vi "Processing Reference (FPGA).vi"() -> ()   [LabVIEW 2019]
uses:
  <vilib>/Platform/TimedLoop/XDataNode/wakeup.ctl
  <vilib>/Platform/TimedLoop/XDataNode/XDNodeRunTimeDep.lvlib
  <vilib>/Platform/TimedLoop/XDataNode/nitl_modes.ctl
  <vilib>/Platform/TimedLoop/XDataNode/timing_clust.ctl
  <vilib>/Platform/TimedLoop/XDataNode/XDataNode.xnode
  <vilib>/eio/EIONode/EIONode.xnode
  <instrlib>/_niInstr/Basic Elements/v1/FPGA/niInstr Basic Elements v1 FPGA.lvlib
  <instrlib>/_niInstr/Data Formatting/v1/FPGA/niInstr Data Formatting v1 FPGA.lvlib
  <vilib>/rvi/DataTransferAndStorage/Container/XNode/niFpgaContainer.xnode
  <vilib>/rvi/FIFO/Fifo_Resource/nirvififoEmulationWrite.vi
  <vilib>/rvi/FIFO/Fifo_Resource/nirvififoEmulationRead.vi
  <vilib>/rvi/LocalResourceManager/LocalResourceManager.xnode
  <vilib>/rvi/FIFO/Fifo_Resource/nirvififoEmulationGetNumberOfElementsToRead.vi
  <vilib>/rvi/interface/RandomDataEmulation/nirviRandomDataFpgaMultiElementTemplate.vi
  <instrlib>/_niInstr/Data Formatting/v1/FPGA/Private/Convert/U8 array to Boolean Array.vi
  <instrlib>/_niInstr/Data Formatting/v1/FPGA/Private/Convert/Boolean Array to U8 Array.vi
  <vilib>/rvi/eio/common/nirviEmuTemplateMethod_errors.vi
  <instrlib>/_niInstr/Basic Elements/v1/FPGA/Private/Count Up U32.vi
  <instrlib>/_niInstr/Basic Elements/v1/FPGA/Private/Count Down U16.vi
  <instrlib>/_niInstr/Basic Elements/v1/FPGA/Private/Count Up U8.vi
  <vilib>/rvi/DataTransferAndStorage/Container/Common/niFpgaContainerGetUniqueNameForEmu.vi
  <vilib>/rvi/DataTransferAndStorage/Container/Common/niFpgaContainerSetEmuInfo.vi
  <vilib>/rvi/eio/common/nirviEmuReportErrorAndStop.vi
  <instrlib>/_niInstr/Instruction Framework/v1/FPGA/Interfaces/Address Space/Address Space Instruction.ctl
  <instrlib>/_niInstr/Instruction Framework/v1/FPGA/Interfaces/Address Space/Address Space.lvclass
  <instrlib>/_niInstr/Instruction Framework/v1/FPGA/Typedefs/Response.ctl
  <instrlib>/_niInstr/Instruction Framework/v1/FPGA/Typedefs/niInstr Instruction Framework v1 FPGA.lvlib
panel:
  out "AXI response out":T1
  out "ready for input":bool
  out "done":bool
  in  "AXI instruction in":T2
  out "channel status":T3(array[cluster])
  out "rx fifo overflow":bool[](array[boolean])
  out "data out port 4":u8[](array[numeric])
  out "data out port 5":u8[](array[numeric])
  in  "data in port 4":u8[](array[numeric])=[0, 0, 0, 0, 0, 0, 0, 0, 0, 0, 0, 0, 0, 0, 0, 0, 0, 0, 0, 0, 0, 0, 0, 0, 0, 0, 0, 0, 0, 0, 0, 0]
  in  "data in port 5":u8[](array[numeric])=[0, 0, 0, 0, 0, 0, 0, 0, 0, 0, 0, 0, 0, 0, 0, 0, 0, 0, 0, 0, 0, 0, 0, 0, 0, 0, 0, 0, 0, 0, 0, 0]
  in  "rx fifo overflow clear":bool
  in  "reset falling edge detect":bool
  out "falling edge detected":bool
  in  "ignore rx fifo prime depth":bool[](array[boolean])=[TRUE, TRUE, TRUE, TRUE, TRUE, TRUE]
  in  "acq length":u16
  in  "software trigger":bool
  in  "data in port 3":u8[](array[numeric])=[0, 0, 0, 0, 0, 0, 0, 0, 0, 0, 0, 0, 0, 0, 0, 0, 0, 0, 0, 0, 0, 0, 0, 0, 0, 0, 0, 0, 0, 0, 0, 0]
  in  "data in port 2":u8[](array[numeric])=[0, 0, 0, 0, 0, 0, 0, 0, 0, 0, 0, 0, 0, 0, 0, 0, 0, 0, 0, 0, 0, 0, 0, 0, 0, 0, 0, 0, 0, 0, 0, 0]
  out "data out port 2":u8[](array[numeric])
  out "data out port 3":u8[](array[numeric])
  in  "tx fifo overflow clear":bool
  out "rx fifo fullness":u32[](array[numeric])
  out "tx fifo overflow":bool[](array[boolean])
  in  "write data":bool
  out "read fifos":bool
  in  "reset read fifo":bool
  in  "rx fifo prime depth":u32=10
  in  "use counter":bool
  in  "data in port 1":u8[](array[numeric])=[0, 0, 0, 0, 0, 0, 0, 0, 0, 0, 0, 0, 0, 0, 0, 0, 0, 0, 0, 0, 0, 0, 0, 0, 0, 0, 0, 0, 0, 0, 0, 0]
  in  "data in port 0":u8[](array[numeric])=[0, 0, 0, 0, 0, 0, 0, 0, 0, 0, 0, 0, 0, 0, 0, 0, 0, 0, 0, 0, 0, 0, 0, 0, 0, 0, 0, 0, 0, 0, 0, 0]
  out "data out port 1":u8[](array[numeric])
  out "data out port 0":u8[](array[numeric])
  out "clocks valid":bool[](array[boolean])
  out "user clk":u32
  out "status.mgt ref clocks locked":bool
  out "status.mgt ref clock valid":bool
  out "status.config complete":bool
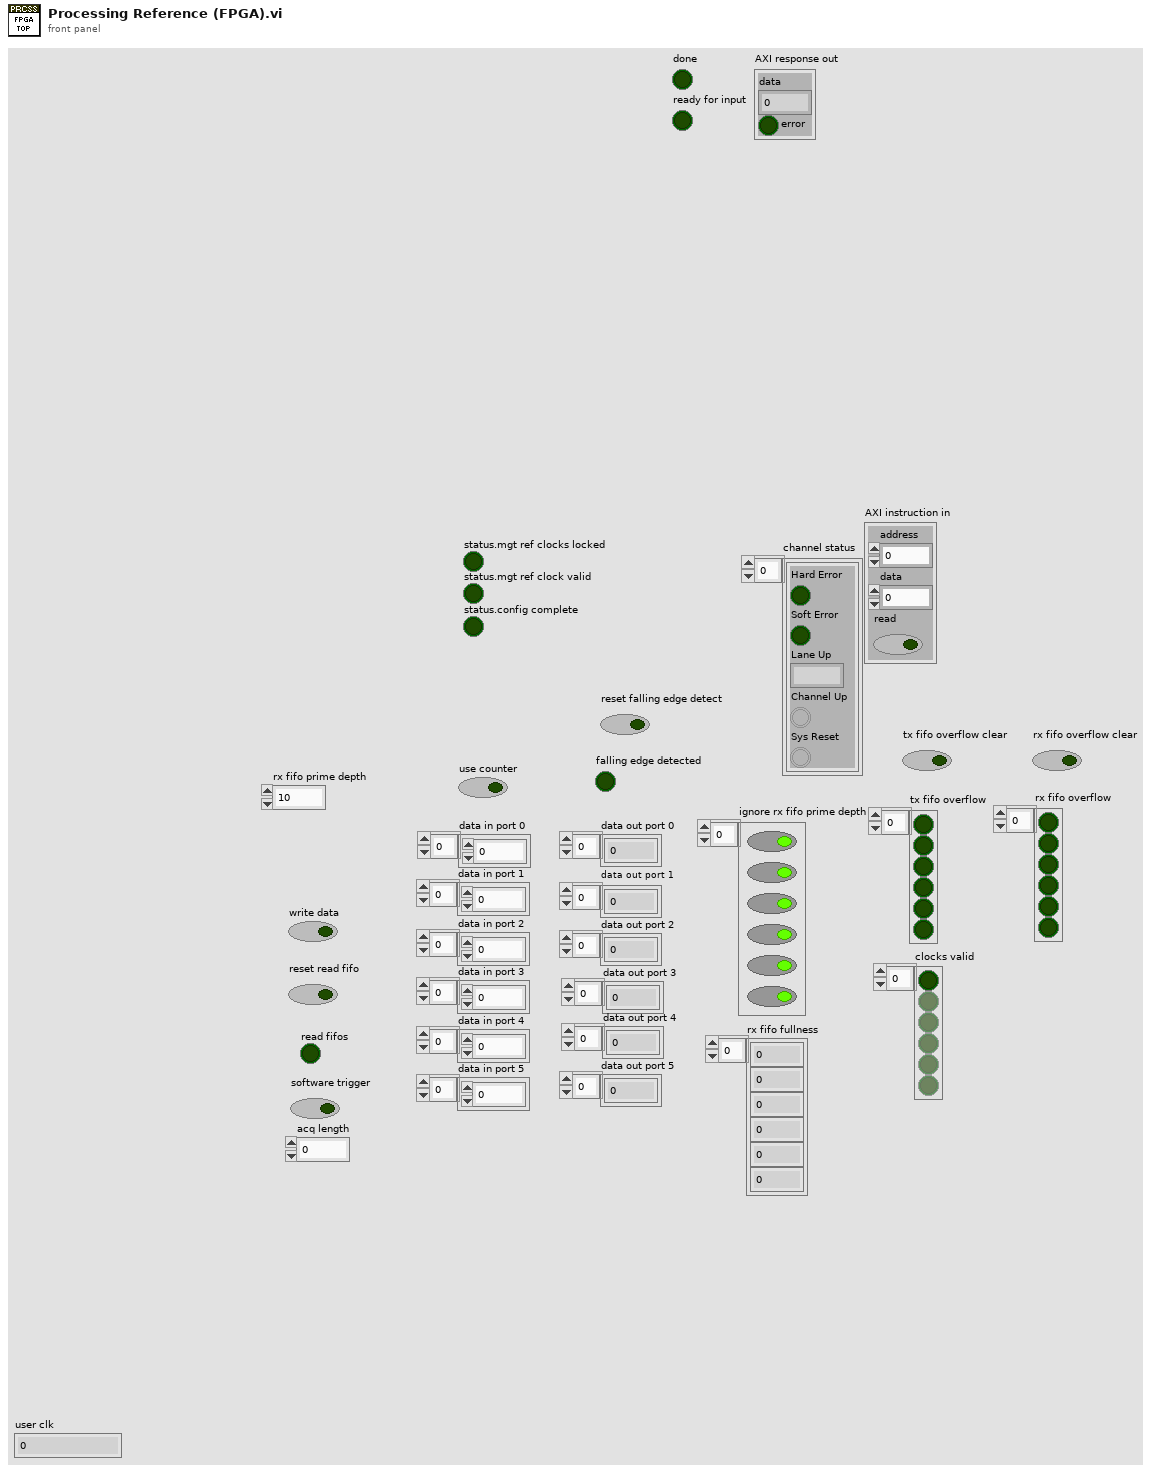
[diagram p1: front panel]
types:
  T1 = typedef "niInstr Instruction Framework v1 FPGA.lvlib/Response.ctl" = cluster{"data":u64, "error":bool}
  T2 = typedef "niInstr Instruction Framework Interfaces v1 FPGA.lvlib/Address Space.lvclass/Address Space Instruction.ctl" = cluster{"address":u32, "data":u64, "read":bool}
  T3 = cluster{"Hard Error":bool, "Soft Error":bool, "Lane Up":fxp<+,4,4>, "Channel Up":bool, "Sys Reset":bool}[]
  T4 = cluster{"m_axis_tvalid":refnum<k21>, "m_axis_tdata_0":refnum<k21>, "m_axis_tdata_1":refnum<k21>, "m_axis_tdata_2":refnum<k21>, "m_axis_tdata_3":refnum<k21>}
  T5 = cluster{"s_axis_tvalid":refnum<k21>, "s_axis_tdata_0":refnum<k21>, "s_axis_tdata_1":refnum<k21>, "s_axis_tdata_2":refnum<k21>, "s_axis_tdata_3":refnum<k21>, "s_axis_tready":refnum<k21>}
  T6 = typedef "XDNodeRunTimeDep.lvlib/timing_clust.ctl" = cluster{"Expected End [f-1]":u64, "Actual End [f-1]":u64, "Finished Late? [f-1]":bool, "Expected End [i-1]":u64, "Actual End [i-1]":u64, "Finished Late? [i-1]":bool, "Expected Start [i]":u64, "Actual Start [i]":u64, "Expected Start [f]":u64, "Actual Start [f]":u64, "Source Name":string, "Structure Name":string, "Period":i64, "Deadline":i64, "Offset":i64, "Start":i64, "Priority":i32, "Timeout":i32, "Mode":T7, "Wakeup Reason":T8, "Error":errorcluster, "Source Type":string, "Secondary Source Type":string, "Global End Time":u64, "Global Start Time":u64, "Frame Duration":u64, "Iteration Duration":u64, "Assigned CPU":i32, "I/O Scan Engine Mode":u32}
  T7 = typedef "XDNodeRunTimeDep.lvlib/nitl_modes.ctl" = enum32{"No Change", "Process missed periods, maintain original phase", "Discard missed periods, maintain original phase", "Process missed periods, ignore original phase", "Discard missed periods, ignore original phase"}
  T8 = typedef "XDNodeRunTimeDep.lvlib/wakeup.ctl" = enum32{"Normal", "Aborted", "Asynchronous wakeup", "Timing source error", "Timed loop error", "Timeout"}
  T9 = typedef "AXI4-Stream Reader FXP64x4 Resources.ctl" = cluster{"AXI4-Stream Reader Resources":cluster{"Use TREADY":bool, "Use TLAST":bool, "TLAST":refnum<k21>, "TREADY":refnum<k21>, "TVALID":refnum<k21>, "Use TKEEP":bool, "Use TSTRB":bool, "Use TUSER":bool}, "TDATA Resources":cluster{"TDATA_0":refnum<k21>, "TDATA_1":refnum<k21>, "TDATA_2":refnum<k21>, "TDATA_3":refnum<k21>}, "TKEEP":refnum<k21>, "TSTRB":refnum<k21>}
  T10 = typedef "AXI4-Stream Writer FXP64x4 Resources.ctl" = cluster{"Writer Resources":cluster{"Use TREADY":bool, "Use TLAST":bool, "TLAST":refnum<k21>, "TREADY":refnum<k21>, "TVALID":refnum<k21>, "Use TSTRB":bool, "Use TKEEP":bool, "Use TUSER":bool}, "TDATA Resources":cluster{"TDATA_0":refnum<k21>, "TDATA_1":refnum<k21>, "TDATA_2":refnum<k21>, "TDATA_3":refnum<k21>}, "TKEEP":refnum<k21>, "TSTRB":refnum<k21>}
  T11 = cluster{"Hard Error":refnum<k21>, "Soft Error":refnum<k21>, "Lane Up":refnum<k21>, "Channel Up":refnum<k21>, "Sys Reset":refnum<k21>}
  T12 = cluster{"Hard Error":bool, "Soft Error":bool, "Lane Up":fxp<+,4,4>, "Channel Up":bool, "Sys Reset":bool}
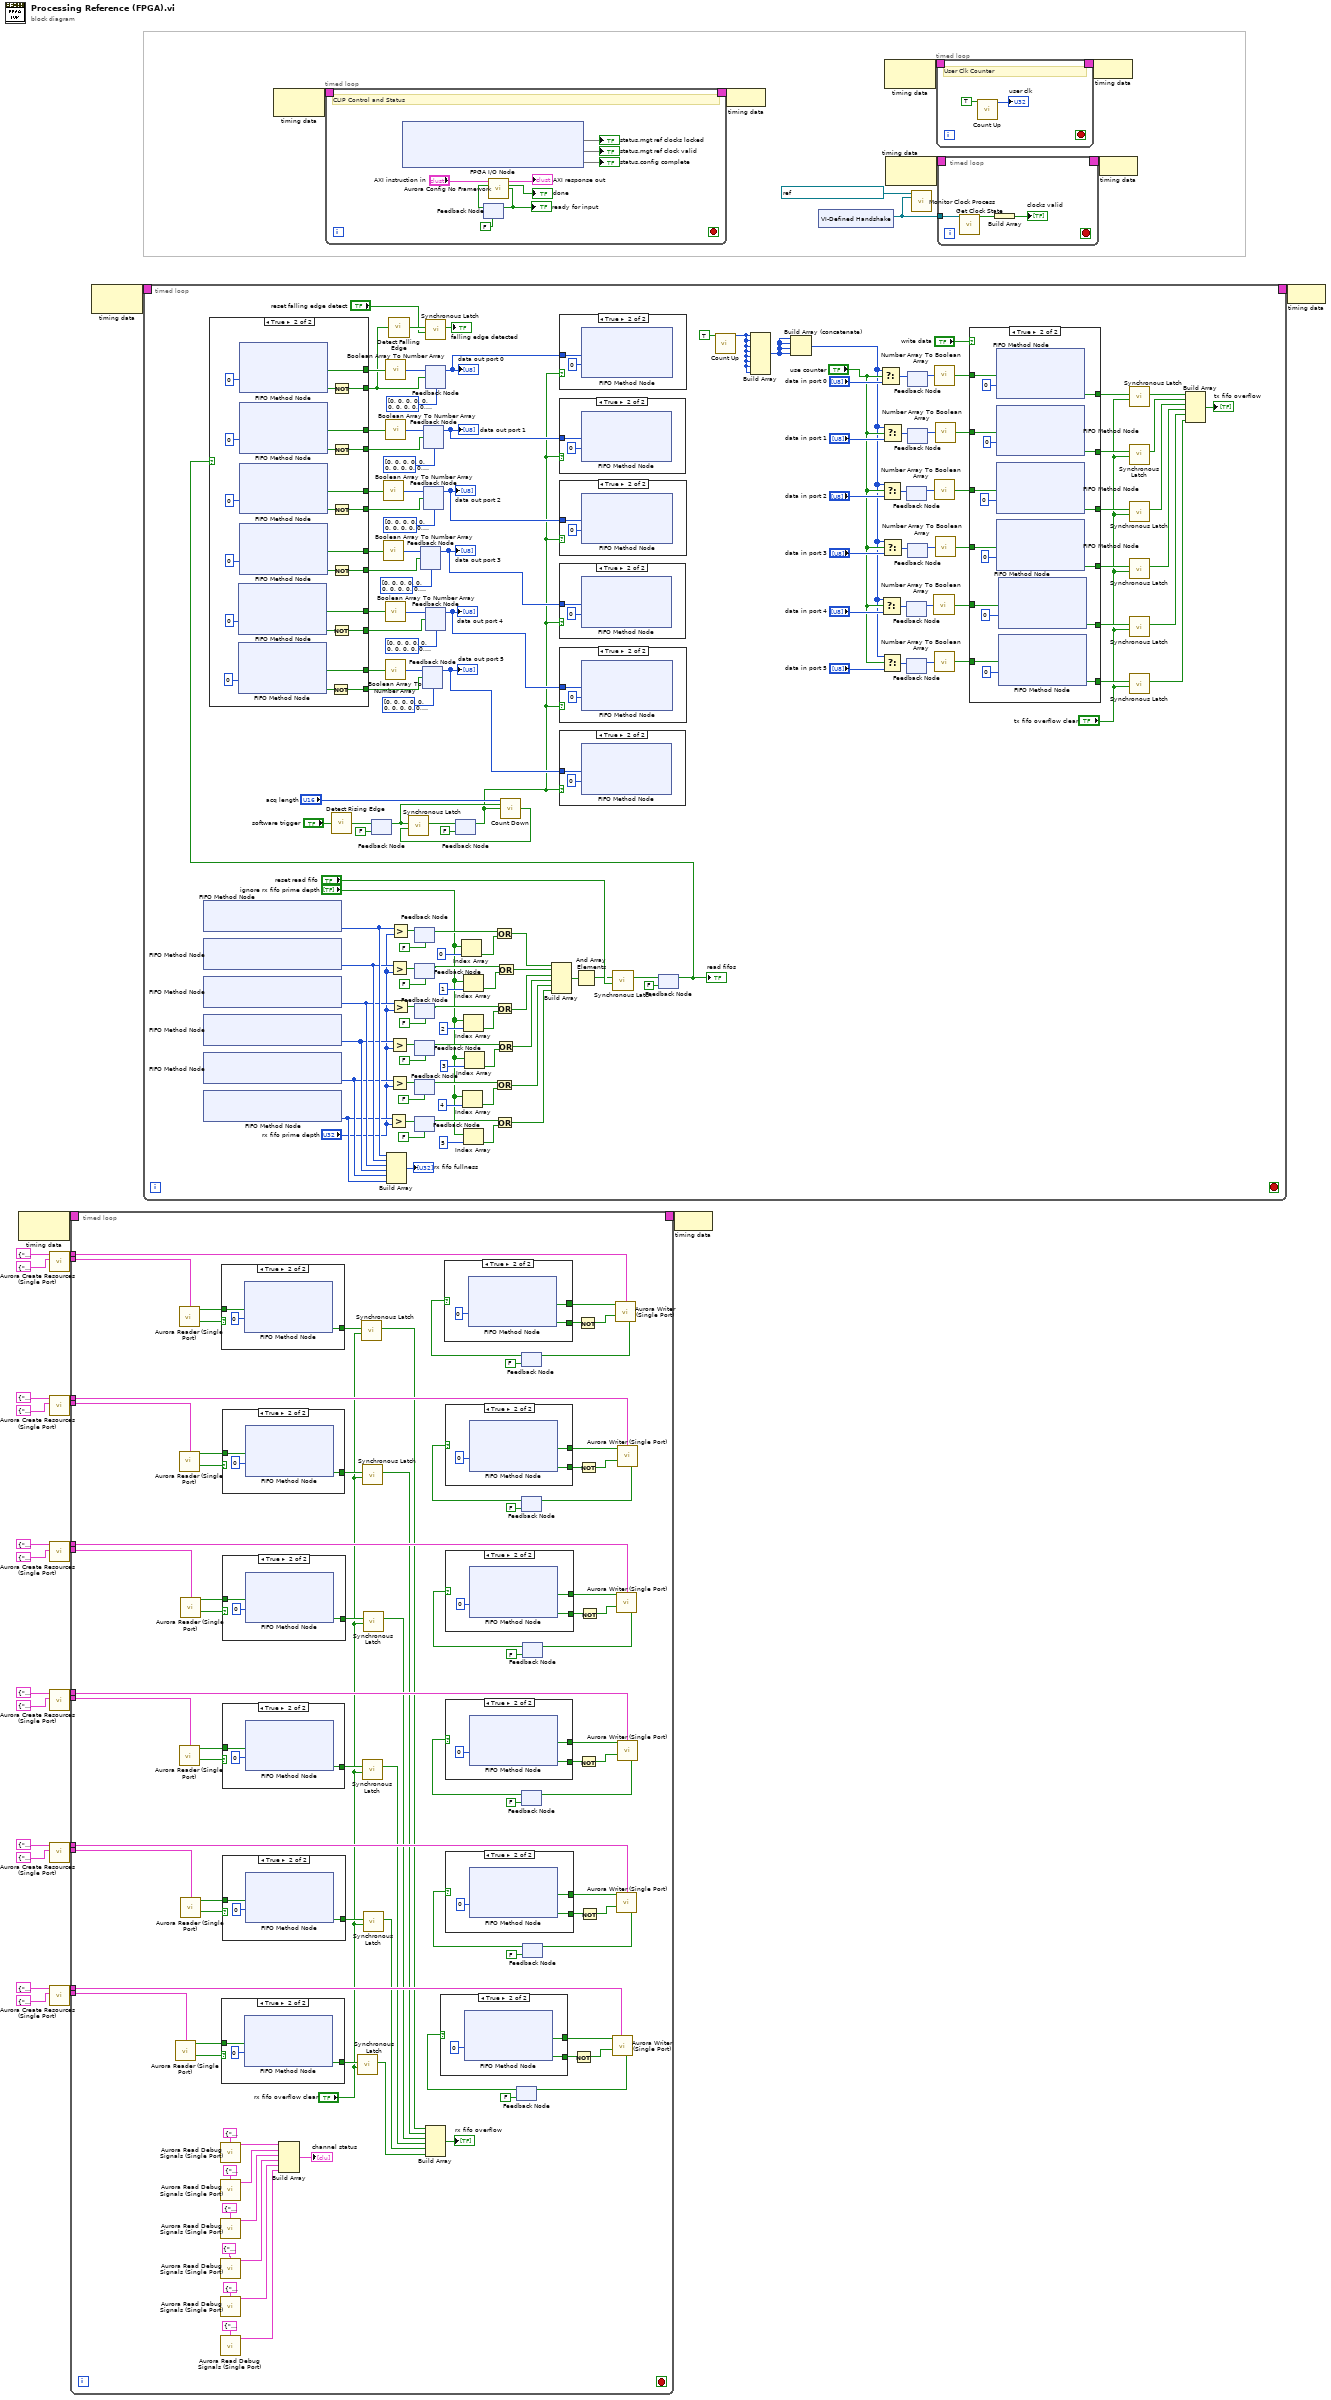
[diagram p0: block diagram]
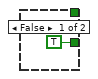
[diagram p2: hidden frame]
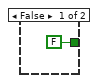
[diagram p3: hidden frame]
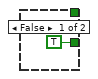
[diagram p4: hidden frame]
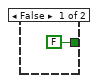
[diagram p5: hidden frame]
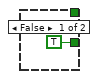
[diagram p6: hidden frame]
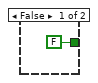
[diagram p7: hidden frame]
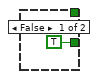
[diagram p8: hidden frame]
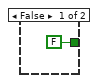
[diagram p9: hidden frame]
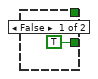
[diagram p10: hidden frame]
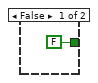
[diagram p11: hidden frame]
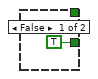
[diagram p12: hidden frame]
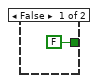
[diagram p13: hidden frame]
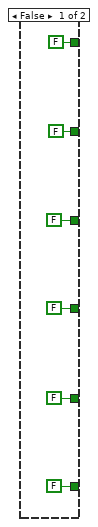
[diagram p20: hidden frame]
diagram:
  n1 = node-c288() -> (w22:T6)  [unwired: 1 in]
  n2 = call "Aurora Create Resources (Single Port).vi"("RX CLIP Resources"=T4 {"m_axis_tvalid"="7902R IO Socket\\uPort0_m_axi_rx_tvalid", "m_axis_tdata_0"="7902R IO Socket\\uPort0_m_axi_rx_tdata_0", "m_axis_tdata_1"="7902R IO Socket\\uPort0_m_axi_rx_tdata_1", "m_axis_tdata_2"="7902R IO Socket\\uPort0_m_axi_rx_tdata_2", "m_axis_tdata_3"="7902R IO Socket\\uPort0_m_axi_rx_tdata_3"}, "TX CLIP Resources"=T5 {"s_axis_tvalid"="7902R IO Socket\\uPort0_s_axi_tx_tvalid", "s_axis_tdata_0"="7902R IO Socket\\uPort0_s_axi_tx_tdata_0", "s_axis_tdata_1"="7902R IO Socket\\uPort0_s_axi_tx_tdata_1", "s_axis_tdata_2"="7902R IO Socket\\uPort0_s_axi_tx_tdata_2", "s_axis_tdata_3"="7902R IO Socket\\uPort0_s_axi_tx_tdata_3", "s_axis_tready"="7902R IO Socket\\uPort0_s_axi_tx_tready"}) -> ("AXI4-Stream Reader FXP64x4"=w20:T9, "AXI4-Stream Writer FXP64x4"=w19:T10)  [unwired: 8 in]
  n3 = call "Aurora Create Resources (Single Port).vi"("RX CLIP Resources"=T4 {"m_axis_tvalid"="7902R IO Socket\\uPort1_m_axi_rx_tvalid", "m_axis_tdata_0"="7902R IO Socket\\uPort1_m_axi_rx_tdata_0", "m_axis_tdata_1"="7902R IO Socket\\uPort1_m_axi_rx_tdata_1", "m_axis_tdata_2"="7902R IO Socket\\uPort1_m_axi_rx_tdata_2", "m_axis_tdata_3"="7902R IO Socket\\uPort1_m_axi_rx_tdata_3"}, "TX CLIP Resources"=T5 {"s_axis_tvalid"="7902R IO Socket\\uPort1_s_axi_tx_tvalid", "s_axis_tdata_0"="7902R IO Socket\\uPort1_s_axi_tx_tdata_0", "s_axis_tdata_1"="7902R IO Socket\\uPort1_s_axi_tx_tdata_1", "s_axis_tdata_2"="7902R IO Socket\\uPort1_s_axi_tx_tdata_2", "s_axis_tdata_3"="7902R IO Socket\\uPort1_s_axi_tx_tdata_3", "s_axis_tready"="7902R IO Socket\\uPort1_s_axi_tx_tready"}) -> ("AXI4-Stream Reader FXP64x4"=w9:T9, "AXI4-Stream Writer FXP64x4"=w10:T10)  [unwired: 8 in]
  n4 = call "Aurora Create Resources (Single Port).vi"("RX CLIP Resources"=T4 {"m_axis_tvalid"="7902R IO Socket\\uPort2_m_axi_rx_tvalid", "m_axis_tdata_0"="7902R IO Socket\\uPort2_m_axi_rx_tdata_0", "m_axis_tdata_1"="7902R IO Socket\\uPort2_m_axi_rx_tdata_1", "m_axis_tdata_2"="7902R IO Socket\\uPort2_m_axi_rx_tdata_2", "m_axis_tdata_3"="7902R IO Socket\\uPort2_m_axi_rx_tdata_3"}, "TX CLIP Resources"=T5 {"s_axis_tvalid"="7902R IO Socket\\uPort2_s_axi_tx_tvalid", "s_axis_tdata_0"="7902R IO Socket\\uPort2_s_axi_tx_tdata_0", "s_axis_tdata_1"="7902R IO Socket\\uPort2_s_axi_tx_tdata_1", "s_axis_tdata_2"="7902R IO Socket\\uPort2_s_axi_tx_tdata_2", "s_axis_tdata_3"="7902R IO Socket\\uPort2_s_axi_tx_tdata_3", "s_axis_tready"="7902R IO Socket\\uPort2_s_axi_tx_tready"}) -> ("AXI4-Stream Reader FXP64x4"=w7:T9, "AXI4-Stream Writer FXP64x4"=w8:T10)  [unwired: 8 in]
  n5 = call "Aurora Create Resources (Single Port).vi"("RX CLIP Resources"=T4 {"m_axis_tvalid"="7902R IO Socket\\uPort3_m_axi_rx_tvalid", "m_axis_tdata_0"="7902R IO Socket\\uPort3_m_axi_rx_tdata_0", "m_axis_tdata_1"="7902R IO Socket\\uPort3_m_axi_rx_tdata_1", "m_axis_tdata_2"="7902R IO Socket\\uPort3_m_axi_rx_tdata_2", "m_axis_tdata_3"="7902R IO Socket\\uPort3_m_axi_rx_tdata_3"}, "TX CLIP Resources"=T5 {"s_axis_tvalid"="7902R IO Socket\\uPort3_s_axi_tx_tvalid", "s_axis_tdata_0"="7902R IO Socket\\uPort3_s_axi_tx_tdata_0", "s_axis_tdata_1"="7902R IO Socket\\uPort3_s_axi_tx_tdata_1", "s_axis_tdata_2"="7902R IO Socket\\uPort3_s_axi_tx_tdata_2", "s_axis_tdata_3"="7902R IO Socket\\uPort3_s_axi_tx_tdata_3", "s_axis_tready"="7902R IO Socket\\uPort3_s_axi_tx_tready"}) -> ("AXI4-Stream Reader FXP64x4"=w5:T9, "AXI4-Stream Writer FXP64x4"=w6:T10)  [unwired: 8 in]
  n6 = call "Aurora Create Resources (Single Port).vi"("RX CLIP Resources"=T4 {"m_axis_tvalid"="7902R IO Socket\\uPort4_m_axi_rx_tvalid", "m_axis_tdata_0"="7902R IO Socket\\uPort4_m_axi_rx_tdata_0", "m_axis_tdata_1"="7902R IO Socket\\uPort4_m_axi_rx_tdata_1", "m_axis_tdata_2"="7902R IO Socket\\uPort4_m_axi_rx_tdata_2", "m_axis_tdata_3"="7902R IO Socket\\uPort4_m_axi_rx_tdata_3"}, "TX CLIP Resources"=T5 {"s_axis_tvalid"="7902R IO Socket\\uPort4_s_axi_tx_tvalid", "s_axis_tdata_0"="7902R IO Socket\\uPort4_s_axi_tx_tdata_0", "s_axis_tdata_1"="7902R IO Socket\\uPort4_s_axi_tx_tdata_1", "s_axis_tdata_2"="7902R IO Socket\\uPort4_s_axi_tx_tdata_2", "s_axis_tdata_3"="7902R IO Socket\\uPort4_s_axi_tx_tdata_3", "s_axis_tready"="7902R IO Socket\\uPort4_s_axi_tx_tready"}) -> ("AXI4-Stream Reader FXP64x4"=w3:T9, "AXI4-Stream Writer FXP64x4"=w4:T10)  [unwired: 8 in]
  n7 = call "Aurora Create Resources (Single Port).vi"("RX CLIP Resources"=T4 {"m_axis_tvalid"="7902R IO Socket\\uPort5_m_axi_rx_tvalid", "m_axis_tdata_0"="7902R IO Socket\\uPort5_m_axi_rx_tdata_0", "m_axis_tdata_1"="7902R IO Socket\\uPort5_m_axi_rx_tdata_1", "m_axis_tdata_2"="7902R IO Socket\\uPort5_m_axi_rx_tdata_2", "m_axis_tdata_3"="7902R IO Socket\\uPort5_m_axi_rx_tdata_3"}, "TX CLIP Resources"=T5 {"s_axis_tvalid"="7902R IO Socket\\uPort5_s_axi_tx_tvalid", "s_axis_tdata_0"="7902R IO Socket\\uPort5_s_axi_tx_tdata_0", "s_axis_tdata_1"="7902R IO Socket\\uPort5_s_axi_tx_tdata_1", "s_axis_tdata_2"="7902R IO Socket\\uPort5_s_axi_tx_tdata_2", "s_axis_tdata_3"="7902R IO Socket\\uPort5_s_axi_tx_tdata_3", "s_axis_tready"="7902R IO Socket\\uPort5_s_axi_tx_tready"}) -> ("AXI4-Stream Reader FXP64x4"=w1:T9, "AXI4-Stream Writer FXP64x4"=w2:T10)  [unwired: 8 in]
  n8 = timed-loop {
    timing: w22 -> [_]
    timing-out: [_] -> w21
    tunnel: w19 -> [w123]
    tunnel: w20 -> [w122]
    tunnel: w10 -> [w101]
    tunnel: w9 -> [w100]
    tunnel: w8 -> [w89]
    tunnel: w7 -> [w88]
    tunnel: w6 -> [w77]
    tunnel: w5 -> [w76]
    tunnel: w4 -> [w65]
    tunnel: w3 -> [w64]
    tunnel: w2 -> [w53]
    tunnel: w1 -> [w52]
    stop <- _ stop-if-true
    n9 = call "Aurora Reader (Single Port) .vi"("AXI4-Stream Reader FXP64x4"=w52) -> ("data"=w59:bool[], "output valid"=w60:bool)  [unwired: 13 in]
    n10 = call "Aurora Reader (Single Port) .vi"("AXI4-Stream Reader FXP64x4"=w122) -> ("data"=w120:bool[], "output valid"=w119:bool)  [unwired: 13 in]
    n11 = call "Aurora Reader (Single Port) .vi"("AXI4-Stream Reader FXP64x4"=w100) -> ("data"=w107:bool[], "output valid"=w108:bool)  [unwired: 13 in]
    n12 = call "Aurora Reader (Single Port) .vi"("AXI4-Stream Reader FXP64x4"=w76) -> ("data"=w83:bool[], "output valid"=w84:bool)  [unwired: 13 in]
    n13 = call "Aurora Reader (Single Port) .vi"("AXI4-Stream Reader FXP64x4"=w88) -> ("data"=w91:bool[], "output valid"=w92:bool)  [unwired: 13 in]
    n14 = call "Aurora Reader (Single Port) .vi"("AXI4-Stream Reader FXP64x4"=w64) -> ("data"=w67:bool[], "output valid"=w68:bool)  [unwired: 13 in]
    n15 = call "Aurora Read Debug Signals (Single Port).vi"("Debug CLIP Resources"=T11 {"Hard Error"="7902R IO Socket\\uPort0_HardError", "Soft Error"="7902R IO Socket\\uPort0_SoftError", "Lane Up"="7902R IO Socket\\uPort0_LaneUp", "Channel Up"="7902R IO Socket\\uPort0_ChannelUp", "Sys Reset"="7902R IO Socket\\uPort0_sys_reset_out"}) -> ("Debug Info"=w43:T12)  [unwired: 14 in]
    n16 = call "Aurora Read Debug Signals (Single Port).vi"("Debug CLIP Resources"=T11 {"Hard Error"="7902R IO Socket\\uPort1_HardError", "Soft Error"="7902R IO Socket\\uPort1_SoftError", "Lane Up"="7902R IO Socket\\uPort1_LaneUp", "Channel Up"="7902R IO Socket\\uPort1_ChannelUp", "Sys Reset"="7902R IO Socket\\uPort1_sys_reset_out"}) -> ("Debug Info"=w42:T12)  [unwired: 14 in]
    n17 = call "Aurora Read Debug Signals (Single Port).vi"("Debug CLIP Resources"=T11 {"Hard Error"="7902R IO Socket\\uPort2_HardError", "Soft Error"="7902R IO Socket\\uPort2_SoftError", "Lane Up"="7902R IO Socket\\uPort2_LaneUp", "Channel Up"="7902R IO Socket\\uPort2_ChannelUp", "Sys Reset"="7902R IO Socket\\uPort2_sys_reset_out"}) -> ("Debug Info"=w41:T12)  [unwired: 14 in]
    n18 = call "Aurora Read Debug Signals (Single Port).vi"("Debug CLIP Resources"=T11 {"Hard Error"="7902R IO Socket\\uPort3_HardError", "Soft Error"="7902R IO Socket\\uPort3_SoftError", "Lane Up"="7902R IO Socket\\uPort3_LaneUp", "Channel Up"="7902R IO Socket\\uPort3_ChannelUp", "Sys Reset"="7902R IO Socket\\uPort3_sys_reset_out"}) -> ("Debug Info"=w40:T12)  [unwired: 14 in]
    n19 = call "Aurora Read Debug Signals (Single Port).vi"("Debug CLIP Resources"=T11 {"Hard Error"="7902R IO Socket\\uPort4_HardError", "Soft Error"="7902R IO Socket\\uPort4_SoftError", "Lane Up"="7902R IO Socket\\uPort4_LaneUp", "Channel Up"="7902R IO Socket\\uPort4_ChannelUp", "Sys Reset"="7902R IO Socket\\uPort4_sys_reset_out"}) -> ("Debug Info"=w39:T12)  [unwired: 14 in]
    n20 = call "Aurora Read Debug Signals (Single Port).vi"("Debug CLIP Resources"=T11 {"Hard Error"="7902R IO Socket\\uPort5_HardError", "Soft Error"="7902R IO Socket\\uPort5_SoftError", "Lane Up"="7902R IO Socket\\uPort5_LaneUp", "Channel Up"="7902R IO Socket\\uPort5_ChannelUp", "Sys Reset"="7902R IO Socket\\uPort5_sys_reset_out"}) -> ("Debug Info"=w38:T12)  [unwired: 14 in]
    n21 = case shown="True" w119 {
      tunnel: w120 -> [_ w171]
      tunnel: [FALSE ("Timed Out?") w169] -> w118
      frame False {
      }
      frame True {
        n22 = xnode ("FIFO Method Node")("Element"=w171, "Timeout"=0) -> ("Timed Out?"=w169:bool)  [unwired: 1 in, 1 out]
      }
    }
    n23 = case shown="True" w60 {
      tunnel: w59 -> [_ w131]
      tunnel: [FALSE ("Timed Out?") w129] -> w55
      frame False {
      }
      frame True {
        n24 = xnode ("FIFO Method Node")("Element"=w131, "Timeout"=0) -> ("Timed Out?"=w129:bool)  [unwired: 1 in, 1 out]
      }
    }
    n25 = case shown="True" w108 {
      tunnel: w107 -> [_ w163]
      tunnel: [FALSE ("Timed Out?") w161] -> w103
      frame False {
      }
      frame True {
        n26 = xnode ("FIFO Method Node")("Element"=w163, "Timeout"=0) -> ("Timed Out?"=w161:bool)  [unwired: 1 in, 1 out]
      }
    }
    n27 = case shown="True" w84 {
      tunnel: w83 -> [_ w147]
      tunnel: [FALSE ("Timed Out?") w145] -> w79
      frame False {
      }
      frame True {
        n28 = xnode ("FIFO Method Node")("Element"=w147, "Timeout"=0) -> ("Timed Out?"=w145:bool)  [unwired: 1 in, 1 out]
      }
    }
    n29 = case shown="True" w92 {
      tunnel: w91 -> [_ w155]
      tunnel: [FALSE ("Timed Out?") w153] -> w93
      frame False {
      }
      frame True {
        n30 = xnode ("FIFO Method Node")("Element"=w155, "Timeout"=0) -> ("Timed Out?"=w153:bool)  [unwired: 1 in, 1 out]
      }
    }
    n31 = case shown="True" w68 {
      tunnel: w67 -> [_ w139]
      tunnel: [FALSE ("Timed Out?") w137] -> w69
      frame False {
      }
      frame True {
        n32 = xnode ("FIFO Method Node")("Element"=w139, "Timeout"=0) -> ("Timed Out?"=w137:bool)  [unwired: 1 in, 1 out]
      }
    }
    n33 = Build Array(w43, w42, w41, w40, w39, w38) -> (→"channel status":T3)
    n34 = call <instrlib>:"Synchronous Latch.vi"("clear"="rx fifo overflow clear", "set"=w55) -> ("out"=w44:bool)  [unwired: 9 in]
    n35 = call <instrlib>:"Synchronous Latch.vi"("clear"="rx fifo overflow clear", "set"=w118) -> ("out"=w49:bool)  [unwired: 9 in]
    n36 = call <instrlib>:"Synchronous Latch.vi"("clear"="rx fifo overflow clear", "set"=w103) -> ("out"=w48:bool)  [unwired: 9 in]
    n37 = call <instrlib>:"Synchronous Latch.vi"("clear"="rx fifo overflow clear", "set"=w79) -> ("out"=w46:bool)  [unwired: 9 in]
    n38 = call <instrlib>:"Synchronous Latch.vi"("clear"="rx fifo overflow clear", "set"=w93) -> ("out"=w47:bool)  [unwired: 9 in]
    n39 = call <instrlib>:"Synchronous Latch.vi"("clear"="rx fifo overflow clear", "set"=w69) -> ("out"=w45:bool)  [unwired: 9 in]
    n40 = Build Array(w49, w48, w47, w46, w45, w44) -> (→"rx fifo overflow":bool[])
    n41 = feedback #1(FALSE ("ready for input")) -> (w57:bool)
    n42 = case shown="True" w57 {
      tunnel: [_ w127] -> w61
      tunnel: [TRUE ("Timed Out?") w126] -> w56
      frame False {
      }
      frame True {
        n43 = xnode ("FIFO Method Node")("Timeout"=0) -> ("Element"=w127:bool[], "Timed Out?"=w126:bool)  [unwired: 1 in, 1 out]
      }
    }
    n44 = feedback #2(FALSE ("ready for input")) -> (w114:bool)
    n45 = case shown="True" w114 {
      tunnel: [_ w167] -> w121
      tunnel: [TRUE ("Timed Out?") w166] -> w117
      frame False {
      }
      frame True {
        n46 = xnode ("FIFO Method Node")("Timeout"=0) -> ("Element"=w167:bool[], "Timed Out?"=w166:bool)  [unwired: 1 in, 1 out]
      }
    }
    n47 = feedback #3(FALSE ("ready for input")) -> (w105:bool)
    n48 = case shown="True" w105 {
      tunnel: [_ w159] -> w109
      tunnel: [TRUE ("Timed Out?") w158] -> w104
      frame False {
      }
      frame True {
        n49 = xnode ("FIFO Method Node")("Timeout"=0) -> ("Element"=w159:bool[], "Timed Out?"=w158:bool)  [unwired: 1 in, 1 out]
      }
    }
    n50 = feedback #4(FALSE ("ready for input")) -> (w81:bool)
    n51 = case shown="True" w81 {
      tunnel: [_ w143] -> w85
      tunnel: [TRUE ("Timed Out?") w142] -> w80
      frame False {
      }
      frame True {
        n52 = xnode ("FIFO Method Node")("Timeout"=0) -> ("Element"=w143:bool[], "Timed Out?"=w142:bool)  [unwired: 1 in, 1 out]
      }
    }
    n53 = feedback #5(FALSE ("ready for input")) -> (w97:bool)
    n54 = case shown="True" w97 {
      tunnel: [_ w151] -> w90
      tunnel: [TRUE ("Timed Out?") w150] -> w94
      frame False {
      }
      frame True {
        n55 = xnode ("FIFO Method Node")("Timeout"=0) -> ("Element"=w151:bool[], "Timed Out?"=w150:bool)  [unwired: 1 in, 1 out]
      }
    }
    n56 = feedback #6(FALSE ("ready for input")) -> (w73:bool)
    n57 = case shown="True" w73 {
      tunnel: [_ w135] -> w66
      tunnel: [TRUE ("Timed Out?") w134] -> w70
      frame False {
      }
      frame True {
        n58 = xnode ("FIFO Method Node")("Timeout"=0) -> ("Element"=w135:bool[], "Timed Out?"=w134:bool)  [unwired: 1 in, 1 out]
      }
    }
    n59 = Not(x=w56) -> (.not. x?=w62:bool)
    n60 = Not(x=w117) -> (.not. x?=w116:bool)
    n61 = Not(x=w104) -> (.not. x?=w110:bool)
    n62 = Not(x=w80) -> (.not. x?=w86:bool)
    n63 = Not(x=w94) -> (.not. x?=w95:bool)
    n64 = Not(x=w70) -> (.not. x?=w71:bool)
    n65 = call "Aurora Writer (Single Port).vi"("input data"=w61, "AXI4-Stream Writer FXP64x4"=w53, "input valid"=w62) -> ("ready for input"=w63:bool)  [unwired: 12 in]
    n66 = feedback-in #1(w63) -> ()
    n67 = call "Aurora Writer (Single Port).vi"("input data"=w121, "AXI4-Stream Writer FXP64x4"=w123, "input valid"=w116) -> ("ready for input"=w115:bool)  [unwired: 12 in]
    n68 = feedback-in #2(w115) -> ()
    n69 = call "Aurora Writer (Single Port).vi"("input data"=w90, "AXI4-Stream Writer FXP64x4"=w89, "input valid"=w95) -> ("ready for input"=w96:bool)  [unwired: 12 in]
    n70 = feedback-in #5(w96) -> ()
    n71 = call "Aurora Writer (Single Port).vi"("input data"=w66, "AXI4-Stream Writer FXP64x4"=w65, "input valid"=w71) -> ("ready for input"=w72:bool)  [unwired: 12 in]
    n72 = feedback-in #6(w72) -> ()
    n73 = call "Aurora Writer (Single Port).vi"("input data"=w109, "AXI4-Stream Writer FXP64x4"=w101, "input valid"=w110) -> ("ready for input"=w111:bool)  [unwired: 12 in]
    n74 = feedback-in #3(w111) -> ()
    n75 = call "Aurora Writer (Single Port).vi"("input data"=w85, "AXI4-Stream Writer FXP64x4"=w77, "input valid"=w86) -> ("ready for input"=w87:bool)  [unwired: 12 in]
    n76 = feedback-in #4(w87) -> ()
  }
  n77 = node-c288() -> (w28:T6)  [unwired: 1 in]
  n78 = timed-loop {
    timing: w28 -> [_]
    timing-out: [_] -> w27
    stop <- _ stop-if-true
    n79 = xnode ("FIFO Method Node")() -> ("Number of Elements to Read"=w287:u32)  [unwired: 1 in, 1 out]
    n80 = xnode ("FIFO Method Node")() -> ("Number of Elements to Read"=w286:u32)  [unwired: 1 in, 1 out]
    n81 = xnode ("FIFO Method Node")() -> ("Number of Elements to Read"=w248:u32)  [unwired: 1 in, 1 out]
    n82 = xnode ("FIFO Method Node")() -> ("Number of Elements to Read"=w247:u32)  [unwired: 1 in, 1 out]
    n83 = xnode ("FIFO Method Node")() -> ("Number of Elements to Read"=w188:u32)  [unwired: 1 in, 1 out]
    n84 = xnode ("FIFO Method Node")() -> ("Number of Elements to Read"=w187:u32)  [unwired: 1 in, 1 out]
    n85 = call <instrlib>:"Detect Rising Edge.vi"("signal"="software trigger") -> ("edge detected"=w260:bool)  [unwired: 14 in]
    n86 = feedback #7(FALSE ("edge detected")) -> (w259:bool)
    n87 = feedback-in #7(w260) -> ()
    n88 = Build Array(w287, w286, w248, w247, w188, w187) -> (→"rx fifo fullness":u32[])
    n89 = Greater?(x=w187, y="rx fifo prime depth") -> (0:w193:bool)
    n90 = Greater?(x=w286, y="rx fifo prime depth") -> (0:w297:bool)
    n91 = Greater?(x=w247, y="rx fifo prime depth") -> (0:w249:bool)
    n92 = Greater?(x=w188, y="rx fifo prime depth") -> (0:w192:bool)
    n93 = Greater?(x=w287, y="rx fifo prime depth") -> (0:w298:bool)
    n94 = Greater?(x=w248, y="rx fifo prime depth") -> (0:w250:bool)
    n95 = feedback #8(FALSE) -> (w196:bool)
    n96 = feedback-in #8(w192) -> ()
    n97 = feedback #9(FALSE) -> (w199:bool)
    n98 = feedback-in #9(w193) -> ()
    n99 = feedback #10(FALSE) -> (w246:bool)
    n100 = feedback-in #10(w298) -> ()
    n101 = feedback #11(FALSE) -> (w241:bool)
    n102 = feedback-in #11(w297) -> ()
    n103 = feedback #12(FALSE) -> (w238:bool)
    n104 = feedback-in #12(w250) -> ()
    n105 = feedback #13(FALSE) -> (w235:bool)
    n106 = feedback-in #13(w249) -> ()
    n107 = feedback #14(u8[] [0, 0, 0, 0, 0, 0, 0, 0, 0, 0, 0, 0, 0, 0, 0, 0, 0, 0, 0, 0, 0, 0, 0, 0, 0, 0, 0, 0, 0, 0, 0, 0] ("data out")) -> (w175:u8[])
    "data out port 3" <- w175
    n108 = feedback #15(u8[] [0, 0, 0, 0, 0, 0, 0, 0, 0, 0, 0, 0, 0, 0, 0, 0, 0, 0, 0, 0, 0, 0, 0, 0, 0, 0, 0, 0, 0, 0, 0, 0] ("data out")) -> (w176:u8[])
    "data out port 5" <- w176
    n109 = feedback #16(u8[] [0, 0, 0, 0, 0, 0, 0, 0, 0, 0, 0, 0, 0, 0, 0, 0, 0, 0, 0, 0, 0, 0, 0, 0, 0, 0, 0, 0, 0, 0, 0, 0] ("data out")) -> (w252:u8[])
    "data out port 1" <- w252
    n110 = feedback #17(u8[] [0, 0, 0, 0, 0, 0, 0, 0, 0, 0, 0, 0, 0, 0, 0, 0, 0, 0, 0, 0, 0, 0, 0, 0, 0, 0, 0, 0, 0, 0, 0, 0] ("data out")) -> (w255:u8[])
    "data out port 2" <- w255
    n111 = feedback #18(u8[] [0, 0, 0, 0, 0, 0, 0, 0, 0, 0, 0, 0, 0, 0, 0, 0, 0, 0, 0, 0, 0, 0, 0, 0, 0, 0, 0, 0, 0, 0, 0, 0] ("data out")) -> (w177:u8[])
    "data out port 4" <- w177
    n112 = feedback #19(u8[] [0, 0, 0, 0, 0, 0, 0, 0, 0, 0, 0, 0, 0, 0, 0, 0, 0, 0, 0, 0, 0, 0, 0, 0, 0, 0, 0, 0, 0, 0, 0, 0] ("data out")) -> (w253:u8[])
    "data out port 0" <- w253
    n113 = feedback #20(FALSE ("out")) -> (w174:bool)
    n114 = Index Array(array="ignore rx fifo prime depth", index=0) -> (element=w244:bool)
    n115 = Index Array(array="ignore rx fifo prime depth", index=4) -> (element=w195:bool)
    n116 = Index Array(array="ignore rx fifo prime depth", index=1) -> (element=w242:bool)
    n117 = Index Array(array="ignore rx fifo prime depth", index=2) -> (element=w239:bool)
    n118 = Index Array(array="ignore rx fifo prime depth", index=5) -> (element=w198:bool)
    n119 = Index Array(array="ignore rx fifo prime depth", index=3) -> (element=w236:bool)
    n120 = Or(x=w246, y=w244) -> (x .or. y?=w230:bool)
    n121 = Or(x=w196, y=w195) -> (x .or. y?=w190:bool)
    n122 = Or(x=w238, y=w239) -> (x .or. y?=w233:bool)
    n123 = Or(x=w199, y=w198) -> (x .or. y?=w189:bool)
    n124 = Or(x=w235, y=w236) -> (x .or. y?=w231:bool)
    n125 = Or(x=w241, y=w242) -> (x .or. y?=w234:bool)
    n126 = call-poly <instrlib>:"Count Down.vi"("count in"="acq length", "load"=w259, "decrement"=w174) -> ("terminal count"=w263:bool)  [unwired: 11 in, 1 out]
    n127 = call <instrlib>:"Synchronous Latch.vi"("clear"=w263, "set"=w259) -> ("out"=w261:bool)  [unwired: 9 in]
    n128 = feedback-in #20(w261) -> ()
    n129 = Build Array(w230, w234, w233, w231, w190, w189) -> (w232:bool[])
    n130 = case shown="True" w174 {
      tunnel: w252 -> [_ w320]
      frame False {
      }
      frame True {
        n131 = xnode ("FIFO Method Node")("Element"=w320, "Timeout"=0) -> ()  [unwired: 1 in, 2 out]
      }
    }
    n132 = case shown="True" w174 {
      tunnel: w175 -> [_ w316]
      frame False {
      }
      frame True {
        n133 = xnode ("FIFO Method Node")("Element"=w316, "Timeout"=0) -> ()  [unwired: 1 in, 2 out]
      }
    }
    n134 = case shown="True" w174 {
      tunnel: w176 -> [_ w312]
      frame False {
      }
      frame True {
        n135 = xnode ("FIFO Method Node")("Element"=w312, "Timeout"=0) -> ()  [unwired: 1 in, 2 out]
      }
    }
    n136 = case shown="True" w174 {
      tunnel: w253 -> [_ w322]
      frame False {
      }
      frame True {
        n137 = xnode ("FIFO Method Node")("Element"=w322, "Timeout"=0) -> ()  [unwired: 1 in, 2 out]
      }
    }
    n138 = case shown="True" w174 {
      tunnel: w255 -> [_ w318]
      frame False {
      }
      frame True {
        n139 = xnode ("FIFO Method Node")("Element"=w318, "Timeout"=0) -> ()  [unwired: 1 in, 2 out]
      }
    }
    n140 = case shown="True" w174 {
      tunnel: w177 -> [_ w314]
      frame False {
      }
      frame True {
        n141 = xnode ("FIFO Method Node")("Element"=w314, "Timeout"=0) -> ()  [unwired: 1 in, 2 out]
      }
    }
    n142 = And Array Elements(Boolean array=w232) -> (logical AND=w229:bool)
    n143 = call <instrlib>:"Synchronous Latch.vi"("clear"="reset read fifo", "set"=w229) -> ("out"=w296:bool)  [unwired: 9 in]
    n144 = feedback #21(FALSE ("out")) -> (w227:bool)
    "read fifos" <- w227
    n145 = case shown="True" w227 {
      tunnel: [w347 w370] -> w222
      tunnel: [_ w369] -> w310
      tunnel: [w347 w367] -> w284
      tunnel: [_ w366] -> w307
      tunnel: [_ w359] -> w275
      tunnel: [_ w358] -> w274
      tunnel: [w347 w357] -> w272
      tunnel: [w347 w356] -> w273
      tunnel: [_ w351] -> w180
      tunnel: [w347 w350] -> w179
      tunnel: [_ w349] -> w181
      tunnel: [w347 w348] -> w178
      frame False {
        w347 = FALSE ("Timed Out?")
      }
      frame True {
        n146 = xnode ("FIFO Method Node")("Timeout"=0) -> ("Element"=w351:bool[], "Timed Out?"=w352:bool)  [unwired: 1 in, 1 out]
        n147 = xnode ("FIFO Method Node")("Timeout"=0) -> ("Element"=w349:bool[], "Timed Out?"=w355:bool)  [unwired: 1 in, 1 out]
        n148 = xnode ("FIFO Method Node")("Timeout"=0) -> ("Element"=w369:bool[], "Timed Out?"=w371:bool)  [unwired: 1 in, 1 out]
        n149 = xnode ("FIFO Method Node")("Timeout"=0) -> ("Element"=w366:bool[], "Timed Out?"=w368:bool)  [unwired: 1 in, 1 out]
        n150 = xnode ("FIFO Method Node")("Timeout"=0) -> ("Element"=w359:bool[], "Timed Out?"=w360:bool)  [unwired: 1 in, 1 out]
        n151 = xnode ("FIFO Method Node")("Timeout"=0) -> ("Element"=w358:bool[], "Timed Out?"=w361:bool)  [unwired: 1 in, 1 out]
        n152 = Not(x=w352) -> (.not. x?=w350:bool)
        n153 = Not(x=w355) -> (.not. x?=w348:bool)
        n154 = Not(x=w371) -> (.not. x?=w370:bool)
        n155 = Not(x=w368) -> (.not. x?=w367:bool)
        n156 = Not(x=w360) -> (.not. x?=w357:bool)
        n157 = Not(x=w361) -> (.not. x?=w356:bool)
      }
    }
    n158 = call-poly <instrlib>:"Boolean Array To Number Array.vi"("data in"=w275) -> ("data out"=w279:u8[])  [unwired: 14 in]
    n159 = call-poly <instrlib>:"Boolean Array To Number Array.vi"("data in"=w274) -> ("data out"=w278:u8[])  [unwired: 14 in]
    n160 = call-poly <instrlib>:"Boolean Array To Number Array.vi"("data in"=w181) -> ("data out"=w182:u8[])  [unwired: 14 in]
    n161 = call-poly <instrlib>:"Boolean Array To Number Array.vi"("data in"=w180) -> ("data out"=w183:u8[])  [unwired: 14 in]
    n162 = call-poly <instrlib>:"Boolean Array To Number Array.vi"("data in"=w310) -> ("data out"=w254:u8[])  [unwired: 14 in]
    n163 = call-poly <instrlib>:"Boolean Array To Number Array.vi"("data in"=w307) -> ("data out"=w281:u8[])  [unwired: 14 in]
    n164 = call <instrlib>:"Detect Falling Edge.vi"("signal"=w222) -> ("edge detected"=w221:bool)  [unwired: 14 in]
    n165 = feedback-in #14(w278, w273) -> ()
    n166 = feedback-in #15(w183, w179) -> ()
    n167 = feedback-in #16(w281, w284) -> ()
    n168 = feedback-in #17(w279, w272) -> ()
    n169 = feedback-in #18(w182, w178) -> ()
    n170 = call <instrlib>:"Synchronous Latch.vi"("clear"="reset falling edge detect", "set"=w221) -> ("out"=→"falling edge detected":bool)  [unwired: 9 in]
    n171 = feedback-in #19(w254, w222) -> ()
    n172 = feedback-in #21(w296) -> ()
    n173 = call-poly <instrlib>:"Count Up.vi"("increment"=TRUE) -> ("count out"=w305:u8)  [unwired: 14 in]
    n174 = Build Array(w305, w305, w305, w305, w305, w305, w305, w305) -> (w212:u8[])
    n175 = Build Array (concatenate)(w212, w212, w212, w212) -> (w204:u8[])
    n176 = Select(t=w204, s="use counter", f="data in port 0") -> (s? t:f=w302:u8[])
    n177 = Select(t=w204, s="use counter", f="data in port 4") -> (s? t:f=w207:u8[])
    n178 = Select(t=w204, s="use counter", f="data in port 2") -> (s? t:f=w270:u8[])
    n179 = Select(t=w204, s="use counter", f="data in port 5") -> (s? t:f=w210:u8[])
    n180 = Select(t=w204, s="use counter", f="data in port 1") -> (s? t:f=w300:u8[])
    n181 = Select(t=w204, s="use counter", f="data in port 3") -> (s? t:f=w267:u8[])
    n182 = feedback #22() -> (w206:u8[])  [unwired: 1 in]
    n183 = feedback-in #22(w207) -> ()
    n184 = feedback #23() -> (w271:u8[])  [unwired: 1 in]
    n185 = feedback-in #23(w270) -> ()
    n186 = feedback #24() -> (w211:u8[])  [unwired: 1 in]
    n187 = feedback-in #24(w210) -> ()
    n188 = feedback-in #25(w302) -> ()
    n189 = feedback #25() -> (w301:u8[])  [unwired: 1 in]
    n190 = feedback #26() -> (w299:u8[])  [unwired: 1 in]
    n191 = feedback-in #26(w300) -> ()
    n192 = feedback #27() -> (w266:u8[])  [unwired: 1 in]
    n193 = feedback-in #27(w267) -> ()
    n194 = call-poly <instrlib>:"Number Array To Boolean Array.vi"("data in"=w206) -> ("data out"=w203:bool[])  [unwired: 14 in]
    n195 = call-poly <instrlib>:"Number Array To Boolean Array.vi"("data in"=w301) -> ("data out"=w295:bool[])  [unwired: 14 in]
    n196 = call-poly <instrlib>:"Number Array To Boolean Array.vi"("data in"=w271) -> ("data out"=w265:bool[])  [unwired: 14 in]
    n197 = call-poly <instrlib>:"Number Array To Boolean Array.vi"("data in"=w211) -> ("data out"=w202:bool[])  [unwired: 14 in]
    n198 = call-poly <instrlib>:"Number Array To Boolean Array.vi"("data in"=w299) -> ("data out"=w294:bool[])  [unwired: 14 in]
    n199 = call-poly <instrlib>:"Number Array To Boolean Array.vi"("data in"=w266) -> ("data out"=w264:bool[])  [unwired: 14 in]
    n200 = case shown="True" "write data" {
      tunnel: [FALSE ("Timed Out?") w346] -> w309
      tunnel: [FALSE ("Timed Out?") w345] -> w308
      tunnel: w295 -> [_ w344]
      tunnel: w294 -> [_ w343]
      tunnel: w265 -> [_ w338]
      tunnel: w264 -> [_ w337]
      tunnel: [FALSE ("Timed Out?") w336] -> w251
      tunnel: [FALSE ("Timed Out?") w335] -> w293
      tunnel: [FALSE ("Timed Out?") w332] -> w217
      tunnel: [FALSE ("Timed Out?") w331] -> w216
      tunnel: w203 -> [_ w330]
      tunnel: w202 -> [_ w329]
      frame False {
      }
      frame True {
        n201 = xnode ("FIFO Method Node")("Element"=w344, "Timeout"=0) -> ("Timed Out?"=w346:bool)  [unwired: 1 in, 1 out]
        n202 = xnode ("FIFO Method Node")("Element"=w343, "Timeout"=0) -> ("Timed Out?"=w345:bool)  [unwired: 1 in, 1 out]
        n203 = xnode ("FIFO Method Node")("Element"=w338, "Timeout"=0) -> ("Timed Out?"=w335:bool)  [unwired: 1 in, 1 out]
        n204 = xnode ("FIFO Method Node")("Element"=w337, "Timeout"=0) -> ("Timed Out?"=w336:bool)  [unwired: 1 in, 1 out]
        n205 = xnode ("FIFO Method Node")("Element"=w330, "Timeout"=0) -> ("Timed Out?"=w332:bool)  [unwired: 1 in, 1 out]
        n206 = xnode ("FIFO Method Node")("Element"=w329, "Timeout"=0) -> ("Timed Out?"=w331:bool)  [unwired: 1 in, 1 out]
      }
    }
    n207 = call <instrlib>:"Synchronous Latch.vi"("clear"="tx fifo overflow clear", "set"=w309) -> ("out"=w292:bool)  [unwired: 9 in]
    n208 = call <instrlib>:"Synchronous Latch.vi"("clear"="tx fifo overflow clear", "set"=w308) -> ("out"=w291:bool)  [unwired: 9 in]
    n209 = call <instrlib>:"Synchronous Latch.vi"("clear"="tx fifo overflow clear", "set"=w293) -> ("out"=w290:bool)  [unwired: 9 in]
    n210 = call <instrlib>:"Synchronous Latch.vi"("clear"="tx fifo overflow clear", "set"=w251) -> ("out"=w289:bool)  [unwired: 9 in]
    n211 = call <instrlib>:"Synchronous Latch.vi"("clear"="tx fifo overflow clear", "set"=w217) -> ("out"=w214:bool)  [unwired: 9 in]
    n212 = call <instrlib>:"Synchronous Latch.vi"("clear"="tx fifo overflow clear", "set"=w216) -> ("out"=w213:bool)  [unwired: 9 in]
    n213 = Build Array(w292, w291, w290, w289, w214, w213) -> (→"tx fifo overflow":bool[])
  }
  n214 = node-c288() -> (w36:T6)  [unwired: 1 in]
  n215 = timed-loop {
    timing: w36 -> [_]
    timing-out: [_] -> w35
    stop <- _ stop-if-true
    # "CLIP Control and Status"
    n216 = xnode "FPGA I/O Node"() -> ("7902R IO Socket\\MgtRefClks_Locked"=→"status.mgt ref clocks locked", "7902R IO Socket\\MgtRefClks_Valid"=→"status.mgt ref clock valid", "7902R IO Socket\\sFrontEndConfig_Complete"=→"status.config complete")  [unwired: 3 in, 3 out]
    n217 = feedback #28(FALSE ("ready for input")) -> (w376:bool)
    n218 = call "Aurora Config No Framework.vi"("address space.lvclass:address space instruction in"="AXI instruction in", "input valid (instruction)"=w376) -> ("response out"=→"AXI response out":T1, "done"=→"done":bool, "ready for input"=w377:bool)  [unwired: 11 in]
    "ready for input" <- w377
    n219 = feedback-in #28(w377) -> ()
  }
  n220 = node-c288(w21) -> ()
  n221 = node-c288(w35) -> ()
  n222 = xnode "VI-Defined Handshake"() -> ("Handshake Out"=w29:refnum<k21>)
  n223 = node-c288() -> (w34:T6)  [unwired: 1 in]
  n224 = node-c288() -> (w32:T6)  [unwired: 1 in]
  n225 = call "Monitor Clock Process.vi"("clock name"=refnum<k21> "7902R IO Socket\\UserClk", "handshake"=w29) -> ()  [unwired: 14 in]
  n226 = timed-loop {
    timing: w34 -> [_]
    timing-out: [_] -> w33
    stop <- _ stop-if-true
    # "User Clk Counter"
    n227 = call-poly <instrlib>:"Count Up.vi"("increment"=TRUE) -> ("count out"=→"user clk":u32)  [unwired: 14 in]
  }
  n228 = timed-loop {
    timing: w32 -> [_]
    timing-out: [_] -> w31
    tunnel: w29 -> [w391]
    stop <- _ stop-if-true
    n229 = call "Get Clock State.vi"("handshake in"=w391) -> ("clock valid"=w390:bool)  [unwired: 14 in]
    n230 = Build Array(w390) -> (→"clocks valid":bool[])
  }
  n231 = node-c288(w33) -> ()
  n232 = node-c288(w31) -> ()
  n233 = node-c288(w27) -> ()
